vi "Set Cluster AutoResize to Vertical.vi"(8 "error in (no error)":errorcluster, 11 "Cluster in":refnum<vi>) -> (0 "error out":errorcluster, 3 "Cluster out":refnum<vi>)   [LabVIEW 2019, in "gRPC Template Creation Utility.lvlib"]
uses:
  gRPC Template Creation Utility.lvlib
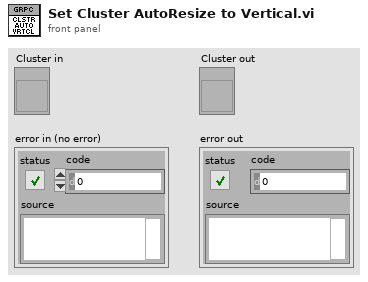
[diagram p1: front panel]
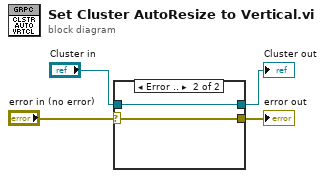
[diagram p0: block diagram]
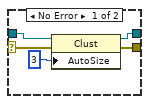
[diagram p2: hidden frame]
diagram:
  n1 = case shown="Error .." "error in (no error)" {
    selector: "error in (no error)" -> [w5 w11]
    tunnel: [w9 w11] -> w4
    tunnel: [w8 w10] -> w3
    tunnel: "Cluster in" -> [w6 w10]
    frame No Error {
      n2 = property class="Clust"(reference=w6, error in=w5, "AutoSize"=u32 3 ("Auto Sizing")) -> (reference out=w8:refnum<vi>, error out=w9:errorcluster)
    }
    frame Error {
    }
  }
  "error out" <- w4
  "Cluster out" <- w3
